vi "version.vi"(7 "LabVIEW Web Service Request":refnum<class "Web Request.lvclass">) -> ()   [LabVIEW 2017]
uses:
  <vilib>/wsapi/Web Request.lvclass
  C:/Program Files (x86)/National Instruments/LabVIEW 2017/vi.lib/wsapi/Web Service.lvclass
  <vilib>/wsapi/Web Service.lvclass
panel:
  # "Use the Web Service Request input terminal to call the VIs on the Web Services palette. Do not remove it from the connector pane unless you don't need access to the palette."
  # "Each additional control wired to the connector pane will be available as an input in the URL. To include an indicator in terminal-mode output (the default setting), it must also be wired to the connector pane."
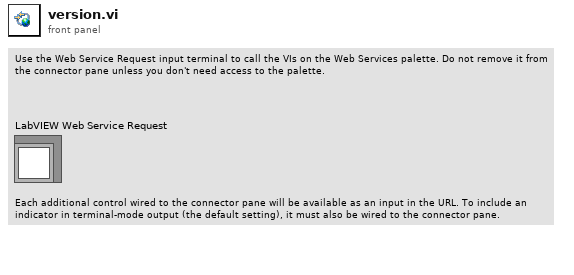
[diagram p1: front panel]
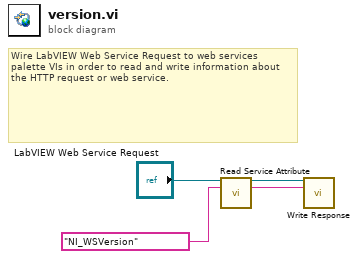
[diagram p0: block diagram]
diagram:
  # "Wire LabVIEW Web Service Request to web services palette VIs in order to read and write information about the HTTP request or web service."
  n1 = call <vilib>:"Read Service Attribute.vi"("LabVIEW Web Service"="LabVIEW Web Service Request", "attribute name"="NI_WSVersion") -> ("LabVIEW Web Service out"=w2:refnum<class "Web Request.lvclass">, "value"=w1:string)  [unwired: 11 in, 1 out]
  n2 = call <vilib>:"Write Response.vi"("LabVIEW Web Service Request"=w2, "response string"=w1) -> ()  [unwired: 12 in, 2 out]
